vi "Slewing Test DAA.vi"(8 "error in (no error)":errorcluster, 10 "Model in":refnum<class "Model.lvclass">, 11 "Test Actuator State in":refnum<class "Test Actuator State.lvclass">) -> (0 "error out":errorcluster, 1 "Pass":bool, 2 "Model out":refnum<class "Model.lvclass">, 3 "Test Actuator State out":refnum<class "Test Actuator State.lvclass">)   [LabVIEW 2016]
uses:
  Model/Model/Model.lvclass
  Typedefs/ActuatorSetPoints.ctl
  <vilib>/Analysis/NI_AALBase.lvlib
  <vilib>/Analysis/baseanly.llb/Mean (DBL).vi
  <vilib>/platform/TimedLoop/XDataNode/XDataNode.xnode
  <vilib>/Platform/TimedLoop/XDataNode/nitl_modes.ctl
  <vilib>/Platform/TimedLoop/XDataNode/XDNodeRunTimeDep.lvlib
  <vilib>/Platform/TimedLoop/XDataNode/wakeup.ctl
  <vilib>/Platform/TimedLoop/XDataNode/timing_clust.ctl
  Model/Waveforms/Waveform/Waveform.lvclass
  Test Actuator State.lvclass
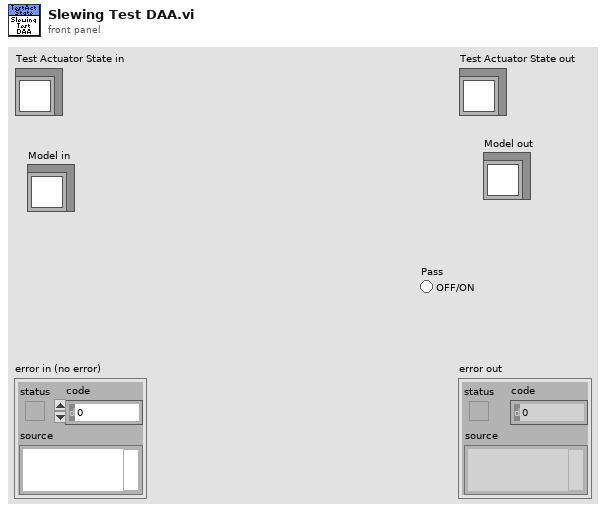
[diagram p1: front panel]
types:
  T1 = typedef "SlewingTestSettings.ctl" = cluster{"Max Force Error (N)":dbl, "Max Moment (NM)":dbl, "Amplitude (N)":dbl, "Max Instance Force Error (N)":dbl, "Ramp Time (s)":dbl, "Hold Time (s)":dbl, "Settling Time (s)":dbl}
  T2 = typedef "XDNodeRunTimeDep.lvlib/timing_clust.ctl" = cluster{"Expected End [f-1]":u64, "Actual End [f-1]":u64, "Finished Late? [f-1]":bool, "Expected End [i-1]":u64, "Actual End [i-1]":u64, "Finished Late? [i-1]":bool, "Expected Start [i]":u64, "Actual Start [i]":u64, "Expected Start [f]":u64, "Actual Start [f]":u64, "Source Name":string, "Structure Name":string, "Period":i64, "Deadline":i64, "Offset":i64, "Start":i64, "Priority":i32, "Timeout":i32, "Mode":T3, "Wakeup Reason":T4, "Error":errorcluster, "Source Type":string, "Secondary Source Type":string, "Global End Time":u64, "Global Start Time":u64, "Frame Duration":u64, "Iteration Duration":u64, "Assigned CPU":i32, "I/O Scan Engine Mode":u32}
  T3 = typedef "XDNodeRunTimeDep.lvlib/nitl_modes.ctl" = enum32{"No Change", "Process missed periods, maintain original phase", "Discard missed periods, maintain original phase", "Process missed periods, ignore original phase", "Discard missed periods, ignore original phase"}
  T4 = typedef "XDNodeRunTimeDep.lvlib/wakeup.ctl" = enum32{"Normal", "Aborted", "Asynchronous wakeup", "Timing source error", "Timed loop error", "Timeout"}
  T5 = typedef "ActuatorSetPoints.ctl" = cluster{"Axial Force":dbl, "Lateral Force":dbl, "FC1 Force":dbl, "FC2 Force":dbl}
  T6 = typedef "ActuatorData.ctl" = cluster{"Timestamp":dbl, "Force":dbl, "Encoder Value":i32}
  T7 = typedef "ToveyEngData.ctl" = cluster{"Timestamp":dbl, "Fx":dbl, "Fy":dbl, "Fz":dbl, "Mx":dbl, "My":dbl, "Mz":dbl}
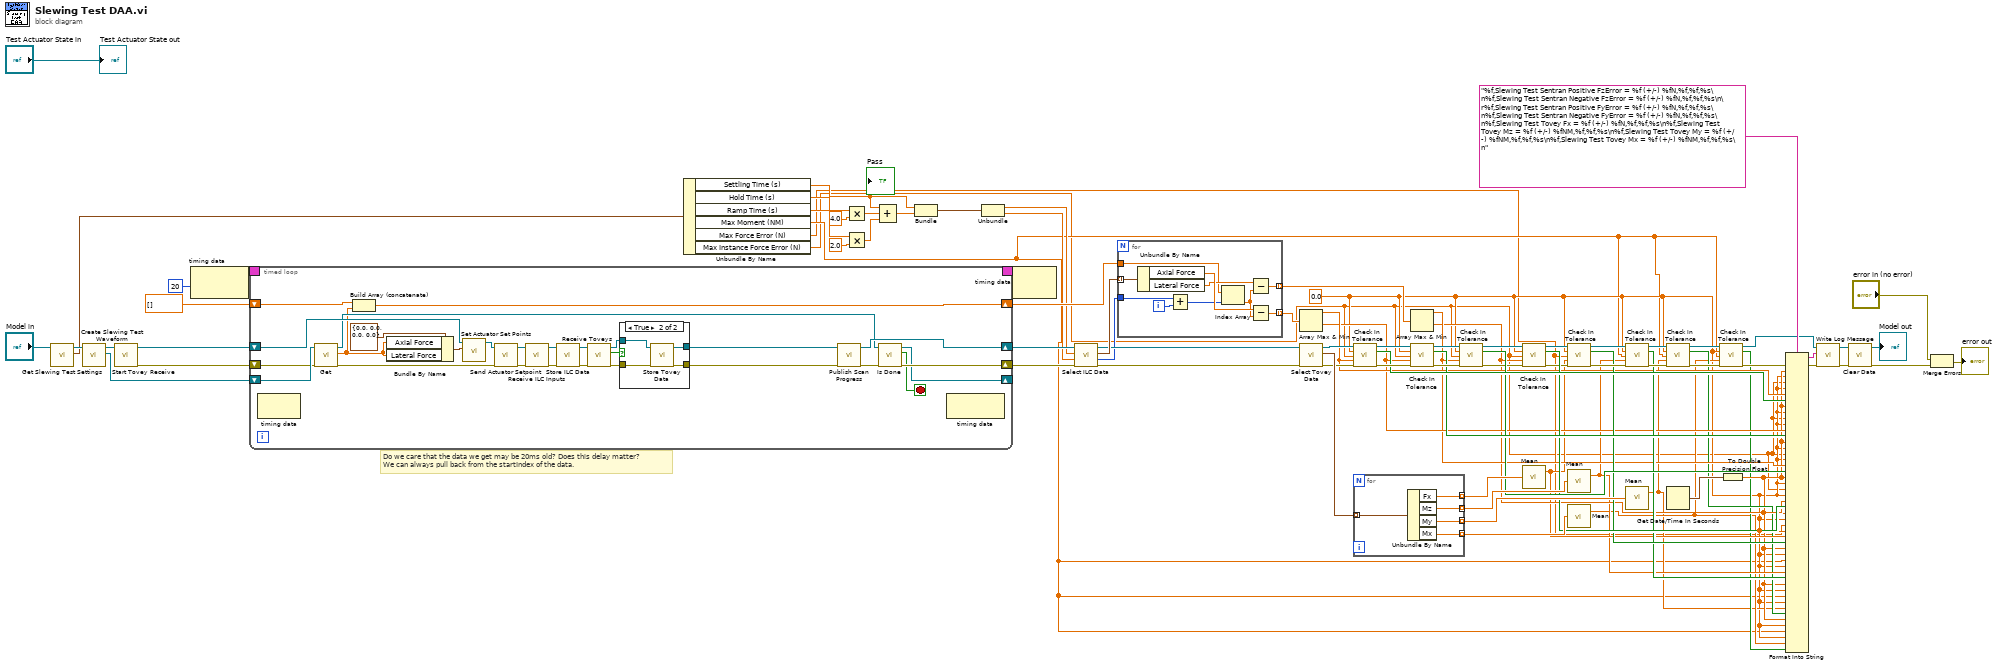
[diagram p0: block diagram]
diagram:
  w6 = 0.0
  # "Do we care that the data we get may be 20ms old? Does this delay matter?\nWe can always pull back from the startIndex of the data."
  n1 = call "Get Slewing Test Settings.vi"("Model in"="Model in") -> ("Slewing Test Settings"=w81:T1, "Model out"=w82:refnum<class "Model.lvclass">)  [unwired: 9 in]
  n2 = call "Create Slewing Test Waveform.vi"("Model in"=w82) -> ("Waveform"=w75:refnum<class "Waveform.lvclass">, "Model out"=w76:refnum<class "Model.lvclass">)  [unwired: 9 in]
  n3 = call "Start Tovey Receive.vi"("Model in"=w76) -> ("error out"=w77:errorcluster, "Model out"=w78:refnum<class "Model.lvclass">)  [unwired: 9 in]
  n4 = node-c288(i64 20 ("Period")) -> (w68:T2)
  n5 = timed-loop {
    shift-right: [w109] -> w74
    shift-left: w78 -> [w101]
    shift-right: [w92] -> w73
    shift-left: w77 -> [w95]
    shift-right: [w90] -> _
    shift-left: w75 -> [w97]
    shift-right: [w87] -> w69
    shift-left: dbl[] [] -> [w89]
    timing: w68 -> [_]
    timing-out: [_] -> w67
    stop <- w91 stop-if-true
    n6 = node-c288() -> ()  [unwired: 1 in, 1 out]
    n7 = call-dynamic "Get.vi"("error in (no error)"=w95, "Waveform in"=w97) -> ("error out"=w94:errorcluster, "Value"=w88:dbl, "Waveform out"=w96:refnum<class "Waveform.lvclass">)  [unwired: 7 in]
    n8 = Build Array (concatenate)(w89, w88) -> (w87:dbl[])
    n9 = Bundle By Name(cluster=T5 {"Axial Force"=0.0, "Lateral Force"=0.0, "FC1 Force"=0.0, "FC2 Force"=0.0} ("Actuator Set Points"), "Axial Force"=w88, "Lateral Force"=w88) -> (w98:T5)
    n10 = call "Set Actuator Set Points.vi"("Actuator Set Points"=w98, "Model in"=w101) -> ("Model out"=w100:refnum<class "Model.lvclass">)  [unwired: 9 in]
    n11 = call "Send Actuator Setpoint.vi"("error in (no error)"=w94, "Model in"=w100) -> ("error out"=w111:errorcluster, "Model out"=w113:refnum<class "Model.lvclass">)  [unwired: 8 in]
    n12 = call "Receive ILC Inputs.vi"("error in (no error)"=w111, "Model in"=w113) -> ("error out"=w110:errorcluster, "Model out"=w112:refnum<class "Model.lvclass">)  [unwired: 8 in]
    n13 = call "Store ILC Data.vi"("error in (no error)"=w110, "Model in"=w112) -> ("error out"=w107:errorcluster, "Model out"=w108:refnum<class "Model.lvclass">)  [unwired: 8 in]
    n14 = call "Receive Toveys.vi"("error in (no error)"=w107, "Model in"=w108) -> ("error out"=w105:errorcluster, "Data Received"=w104:bool, "Model out"=w106:refnum<class "Model.lvclass">)  [unwired: 7 in]
    n15 = case shown="True" w104 {
      tunnel: w106 -> [w117 w121]
      tunnel: w105 -> [w116 w120]
      tunnel: [w116 w119] -> w102
      tunnel: [w117 w118] -> w103
      frame False {
      }
      frame True {
        n16 = call "Store Tovey Data.vi"("error in (no error)"=w120, "Model in"=w121) -> ("error out"=w119:errorcluster, "Model out"=w118:refnum<class "Model.lvclass">)  [unwired: 8 in]
      }
    }
    n17 = call "Publish Scan Progress.vi"("error in (no error)"=w102, "Model in"=w103) -> ("error out"=w93:errorcluster, "Model out"=w109:refnum<class "Model.lvclass">)  [unwired: 8 in]
    n18 = call-dynamic "Is Done.vi"("error in (no error)"=w93, "Waveform in"=w96) -> ("error out"=w92:errorcluster, "Is Done"=w91:bool, "Waveform out"=w90:refnum<class "Waveform.lvclass">)  [unwired: 7 in]
    n19 = node-c288() -> ()  [unwired: 1 in, 1 out]
  }
  n20 = Unbundle By Name(w81) -> ("Settling Time (s)"=w59:dbl, "Hold Time (s)"=w63:dbl, "Ramp Time (s)"=w65:dbl, "Max Moment (NM)"=w3:dbl, "Max Force Error (N)"=w2:dbl, "Max Instance Force Error (N)"=w1:dbl)
  n21 = Multiply(x=w65, y=4.0) -> (x*y=w61:dbl)
  n22 = Multiply(x=w63, y=2.0) -> (x*y=w60:dbl)
  n23 = Compound Arithmetic op=ADD(w59, w61, w60) -> (w58:dbl)
  n24 = Bundle("Settling Time (s)"=w59, w58) -> (w57:cluster{"Settling Time (s)":dbl, dbl})  [unwired: 1 in]
  n25 = Unbundle(w57) -> ("Settling Time (s)"=w5:dbl, w4:dbl)
  n26 = node-c288(w67) -> ()  [unwired: 1 out]
  n27 = call "Select ILC Data.vi"("error in (no error)"=w73, "End Time"=w4, "Start Time"=w5, "Model in"=w74) -> ("error out"=w54:errorcluster, "StartIndex"=w42:i32, "Data"=w56:T6[], "Model out"=w55:refnum<class "Model.lvclass">)  [unwired: 4 in]
  n28 = for {
    tunnel: w56 -> [w131] mode=indexing
    tunnel: [w129] -> w41 mode=indexing
    tunnel: [w127] -> w39 mode=indexing
    tunnel: w69 -> [w123]
    tunnel: w42 -> [w126]
    i -> [w125]
    n29 = Unbundle By Name(w131) -> ("Axial Force"=w130:dbl, "Lateral Force"=w128:dbl)
    n30 = Add(x=w126, y=w125) -> (x+y=w124:i32)
    n31 = Index Array(array=w123, index=w124) -> (element=w122:dbl)
    n32 = Subtract(x=w128, y=w122) -> (x-y=w127:dbl)
    n33 = Subtract(x=w130, y=w122) -> (x-y=w129:dbl)
  }
  n34 = Array Max & Min(array=w41) -> (max value=w17:dbl, min value=w16:dbl)  [unwired: 2 out]
  n35 = call "Select Tovey Data.vi"("error in (no error)"=w54, "Model in"=w55) -> ("error out"=w49:errorcluster, "Data"=w53:T7[], "Model out"=w50:refnum<class "Model.lvclass">)  [unwired: 6 in, 1 out]
  n36 = call "Check In Tolerance.vi"("Model in"=w50, "Expected"=w6, "Tolerance"=w1, "Actual"=w17, "error in (no error)"=w49) -> ("Model out"=w32:refnum<class "Model.lvclass">, "Pass"=w37:bool, "error out"=w40:errorcluster)  [unwired: 8 in]
  n37 = for {
    tunnel: [w136] -> w46 mode=indexing
    tunnel: [w135] -> w45 mode=indexing
    tunnel: [w134] -> w44 mode=indexing
    tunnel: [w133] -> w43 mode=indexing
    tunnel: w53 -> [w132] mode=indexing
    n38 = Unbundle By Name(w132) -> ("Fx"=w136:dbl, "Mz"=w135:dbl, "My"=w134:dbl, "Mx"=w133:dbl)
  }
  n39 = Array Max & Min(array=w39) -> (max value=w15:dbl, min value=w14:dbl)  [unwired: 2 out]
  n40 = call "Check In Tolerance.vi"("Model in"=w32, "Expected"=w6, "Tolerance"=w1, "Actual"=w16, "error in (no error)"=w40) -> ("Model out"=w31:refnum<class "Model.lvclass">, "Pass"=w36:bool, "error out"=w38:errorcluster)  [unwired: 8 in]
  n41 = call "Check In Tolerance.vi"("Model in"=w31, "Expected"=w6, "Tolerance"=w1, "Actual"=w15, "error in (no error)"=w38) -> ("Model out"=w30:refnum<class "Model.lvclass">, "Pass"=w35:bool, "error out"=w34:errorcluster)  [unwired: 8 in]
  n42 = call "Check In Tolerance.vi"("Model in"=w30, "Expected"=w6, "Tolerance"=w1, "Actual"=w14, "error in (no error)"=w34) -> ("Model out"=w19:refnum<class "Model.lvclass">, "Pass"=w33:bool, "error out"=w29:errorcluster)  [unwired: 8 in]
  n43 = call-poly <vilib>:"Mean.vi"("X"=w46) -> ("mean"=w13:dbl)  [unwired: 1 out]
  n44 = call "Check In Tolerance.vi"("Model in"=w19, "Expected"=w6, "Tolerance"=w2, "Actual"=w13, "error in (no error)"=w29) -> ("Model out"=w20:refnum<class "Model.lvclass">, "Pass"=w25:bool, "error out"=w28:errorcluster)  [unwired: 8 in]
  n45 = call-poly <vilib>:"Mean.vi"("X"=w45) -> ("mean"=w12:dbl)  [unwired: 1 out]
  n46 = call-poly <vilib>:"Mean.vi"("X"=w43) -> ("mean"=w8:dbl)  [unwired: 1 out]
  n47 = call "Check In Tolerance.vi"("Model in"=w20, "Expected"=w6, "Tolerance"=w3, "Actual"=w12, "error in (no error)"=w28) -> ("Model out"=w21:refnum<class "Model.lvclass">, "Pass"=w24:bool, "error out"=w27:errorcluster)  [unwired: 8 in]
  n48 = call-poly <vilib>:"Mean.vi"("X"=w44) -> ("mean"=w7:dbl)  [unwired: 1 out]
  n49 = call "Check In Tolerance.vi"("Model in"=w21, "Expected"=w6, "Tolerance"=w3, "Actual"=w7, "error in (no error)"=w27) -> ("Model out"=w22:refnum<class "Model.lvclass">, "Pass"=w11:bool, "error out"=w26:errorcluster)  [unwired: 8 in]
  n50 = Get Date/Time In Seconds() -> (seconds since 1Jan1904=w51:timestamp)
  n51 = call "Check In Tolerance.vi"("Model in"=w22, "Expected"=w6, "Tolerance"=w3, "Actual"=w8, "error in (no error)"=w26) -> ("Model out"=w18:refnum<class "Model.lvclass">, "Pass"=w9:bool, "error out"=w23:errorcluster)  [unwired: 8 in]
  n52 = To Double Precision Float(number=w51) -> (double precision float=w10:dbl)
  n53 = Format Into String(format string="%f,Slewing Test Sentran Positive FzError = %f (+/-) %fN,%f,%f,%s\n%f,Slewing Test Sentran Negative FzError = %f (+/-) %fN,%f,%f,%s\n\r%f,Slewing Test Sentran Positive FyError = %f (+/-) %fN,%f,%f,%s\n%f,Slewing Test Sentran Negative FyError = %f (+/-) %fN,%f,%f,%s\n%f,Slewing Test Tovey Fx = %f (+/-) %fN,%f,%f,%s\n%f,Slewing Test Tovey Mz = %f (+/-) %fNM,%f,%f,%s\n%f,Slewing Test Tovey My = %f (+/-) %fNM,%f,%f,%s\n%f,Slewing Test Tovey Mx = %f (+/-) %fNM,%f,%f,%s\n", error in=w23, w10, w6, w1, w6, w17, w37, w10, w6, w1, w6, w16, w36, w10, w6, w1, w6, w15, w35, w10, w6, w1, w6, w14, w33, w10, w6, w2, w6, w13, w25, w10, w6, w3, w6, w12, w24, w10, w6, w3, w6, w7, w11, w10, w6, w3, w6, w8, w9) -> (resulting string=w47:string, error out=w48:errorcluster)  [unwired: 1 in]
  n54 = call "Write Log Message.vi"("error in (no error)"=w48, "Message"=w47, "Model in"=w18) -> ("error out"=w72:errorcluster, "Model out"=w71:refnum<class "Model.lvclass">)  [unwired: 7 in]
  n55 = call "Clear Data.vi"("error in (no error)"=w72, "Model in"=w71) -> ("error out"=w80:errorcluster, "Model out"=→"Model out":refnum<class "Model.lvclass">)  [unwired: 8 in]
  n56 = Merge Errors("error in (no error)", w80) -> (→"error out":errorcluster)
  "Test Actuator State out" <- "Test Actuator State in"
